vi "fpga_8ch-Main.vi"   [LabVIEW 2011]
uses:
  <vilib>/Platform/TimedLoop/XDataNode/timing_clust.ctl
  <vilib>/Platform/TimedLoop/XDataNode/nitl_modes.ctl
  <vilib>/Platform/TimedLoop/XDataNode/wakeup.ctl
  <vilib>/Platform/TimedLoop/XDataNode/XDataNode.xnode
  <vilib>/Platform/TimedLoop/XDataNode/XDNodeRunTimeDep.lvlib
types:
  T1 = typedef "XDNodeRunTimeDep.lvlib/timing_clust.ctl" = cluster{"Expected End [f-1]":u64, "Actual End [f-1]":u64, "Finished Late? [f-1]":bool, "Expected End [i-1]":u64, "Actual End [i-1]":u64, "Finished Late? [i-1]":bool, "Expected Start [i]":u64, "Actual Start [i]":u64, "Expected Start [f]":u64, "Actual Start [f]":u64, "Source Name":string, "Structure Name":string, "Period":i64, "Deadline":i64, "Offset":i64, "Start":i64, "Priority":i32, "Timeout":i32, "Mode":T2, "Wakeup Reason":T3, "Error":errorcluster, "Source Type":string, "Secondary Source Type":string, "Global End Time":u64, "Global Start Time":u64, "Frame Duration":u64, "Iteration Duration":u64, "Assigned CPU":i32, "I/O Scan Engine Mode":u32}
  T2 = typedef "XDNodeRunTimeDep.lvlib/nitl_modes.ctl" = enum32{"No Change", "Process missed periods, maintain original phase", "Discard missed periods, maintain original phase", "Process missed periods, ignore original phase", "Discard missed periods, ignore original phase"}
  T3 = typedef "XDNodeRunTimeDep.lvlib/wakeup.ctl" = enum32{"Normal", "Aborted", "Asynchronous wakeup", "Timing source error", "Timed loop error", "Timeout"}
  T4 = cluster{"Connector0/DIO0":bool, "Connector0/DIO1":bool, "Connector0/DIO2":bool, "Connector0/DIO3":bool, "Connector0/DIO4":bool, "Connector0/DIO5":bool, "Connector0/DIO6":bool, "Connector0/DIO7":bool}
  T5 = cluster{"D0":bool, "D1":bool, "D2":bool, "D3":bool, "D4":bool, "D5":bool, "D6":bool, "D7":bool}
  T6 = cluster{"D0":u32, "D1 2":u32, "D2 3":u32, "D3 4":u32, "D4 5":u32, "D5 6":u32, "D6 7":u32, "D7 8":u32}
  T7 = typedef "Time Stamp Data.ctl" = cluster{"Timestamp":u32, "Data available":bool}
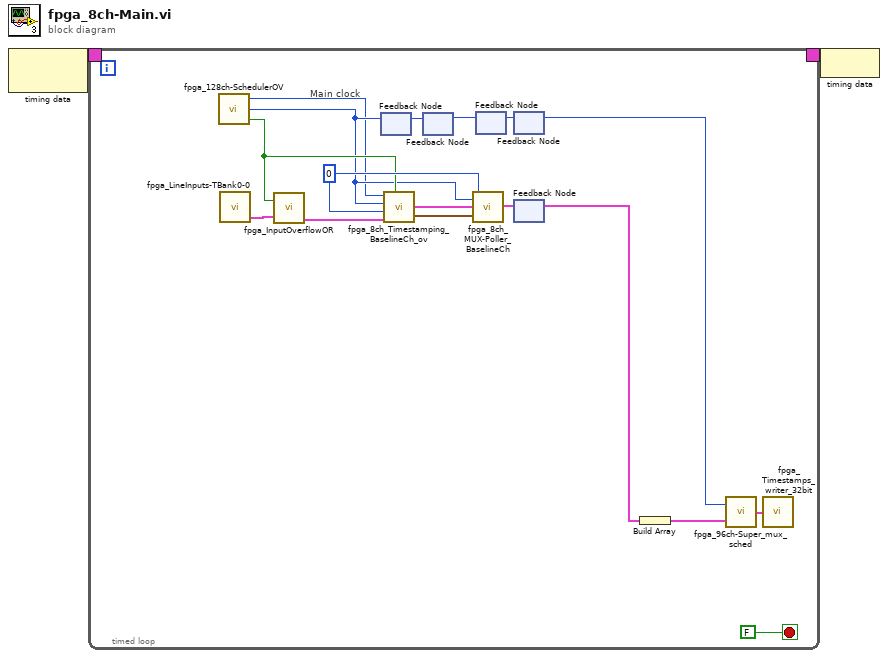
[diagram p0: block diagram]
diagram:
  n1 = node-c288() -> (w2:T1)  [unwired: 1 in]
  n2 = timed-loop {
    timing: w2 -> [_]
    timing-out: [_] -> w1
    stop <- FALSE stop-if-true
    w16 = u8 0 ("Baseline Ch")
    # "Main clock"
    n3 = call "fpga_128ch-SchedulerOV.vi"() -> ("overflow"=w5:bool, "FIFO Schedule"=w4:u8, "Main clock"=w3:u32)  [unwired: 3 in]
    n4 = call "fpga_LineInputs-TBank0-0.vi"() -> ("DataLines"=w12:T4)  [unwired: 5 in]
    n5 = call "fpga_InputOverflowOR.vi"("Input Lines"=w12, "overflow"=w5) -> ("Output Lines"=w10:T4)
    n6 = feedback #1() -> (w9:u8)  [unwired: 1 in]
    n7 = feedback-in #1(w4) -> ()
    n8 = call "fpga_8ch_Timestamping_BaselineCh_ov.vi"("Main clock"=w3, "Scheduler"=w4, "Baseline Ch"=w16, "Signal IN"=w10, "overflow"=w5) -> ("Data available"=w17:T5, "Timestamp bundle"=w18:T6)
    n9 = feedback #2() -> (w8:u8)  [unwired: 1 in]
    n10 = feedback-in #2(w9) -> ()
    n11 = call "fpga_8ch_MUX-Poller_BaselineCh.vi"("Timestamp bundle"=w18, "Data available"=w17, "Scheduler"=w4, "Baseline CH"=w16) -> ("8Ch Timestamps"=w11:T7)
    n12 = feedback #3() -> (w7:u8)  [unwired: 1 in]
    n13 = feedback-in #3(w8) -> ()
    n14 = feedback-in #4(w7) -> ()
    n15 = feedback #4() -> (w6:u8)  [unwired: 1 in]
    n16 = feedback-in #5(w11) -> ()
    n17 = feedback #5() -> (w13:T7)  [unwired: 1 in]
    n18 = Build Array(w13) -> (w15:T7[])
    n19 = call "fpga_96ch-Super_mux_sched.vi"("12 8Ch-timestamp-data array"=w15, "Scheduler"=w6) -> ("All Ch Timestamps"=w14:T7)
    n20 = call "fpga_Timestamps_writer_32bit.vi"("All Ch Timestamps"=w14) -> ()  [unwired: 1 in]
  }
  n21 = node-c288(w1) -> ()
